vi "Shuffled Array (LabVIEW 2021).vi"() -> ()   [LabVIEW 2021]
uses:
  461c6303-d2e4-4249-a56b-5dcc835354f9.vi
panel:
  out "Shuffled Array":dbl[](array[numeric])
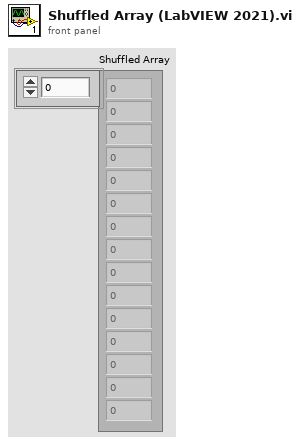
[diagram p1: front panel]
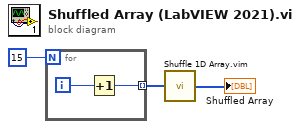
[diagram p0: block diagram]
diagram:
  n1 = for {
    N: 15 -> [_]
    tunnel: [w4] -> w1 mode=indexing
    i -> [w5]
    n2 = Increment(x=w5) -> (x+1=w4:i32)
  }
  n3 = call "Shuffle 1D Array.vim"("array"=w1) -> ("shuffled array"=→"Shuffled Array":i32[])  [unwired: 4 in]
